vi "sv_Compute Time to Next Optimum for Sine Wave.vi"(7 "optimum":T1, 10 "phase (0 °)":dbl, 11 "frequency (997 Hz)":dbl) -> (3 "time to optimum [s]":dbl)   [LabVIEW 2017, in "SoundVib_Generation.lvlib"]
uses:
  <vilib>/addons/_NISVFA/_Generation/SoundVib_Generation.lvlib
  <vilib>/addons/_NISVFA/_Generation/subVIs/sv_Optimum Location.ctl
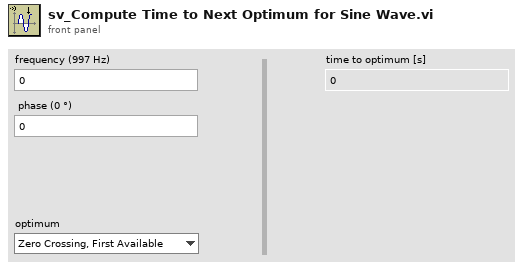
[diagram p1: front panel]
types:
  T1 = typedef "SoundVib_Generation.lvlib/sv_Optimum Location.ctl" = enum16{"Zero Crossing, First Available", "Zero Crossing, Positive Slope", "Zero Crossing, Negative Slope", "Peak or Valley", "Peak", "Valley"}
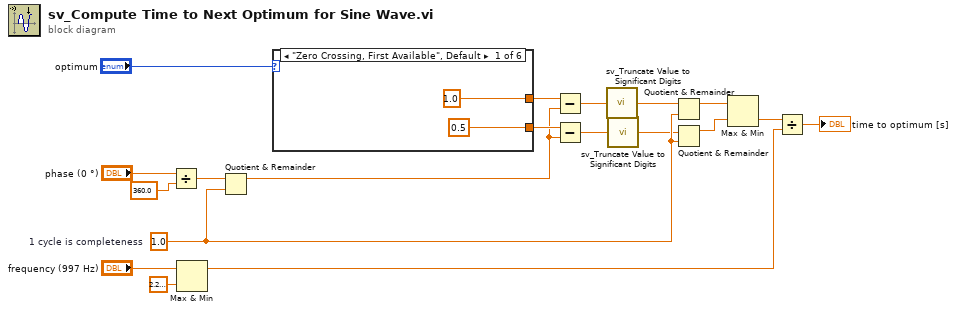
[diagram p0: block diagram]
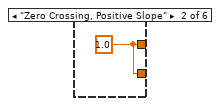
[diagram p2: hidden frame]
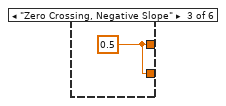
[diagram p3: hidden frame]
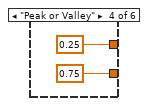
[diagram p4: hidden frame]
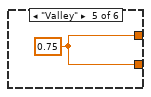
[diagram p5: hidden frame]
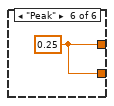
[diagram p6: hidden frame]
diagram:
  w8 = 1.0  # 1 cycle is completeness
  n1 = Divide(x="phase (0 °)", y=360.0 ("time to optimum [s]")) -> (x/y=w16:dbl)
  n2 = Max & Min(x="frequency (997 Hz)", y=2.220446049250313e-16) -> (max(x,y)=w11:dbl)  [unwired: 1 out]
  n3 = Quotient & Remainder(x=w16, y=w8) -> (x-y*floor(x/y)=w6:dbl)  [unwired: 1 out]
  n4 = case shown="\"Zero Crossing, First Available\", Default" "optimum" {
    tunnel: [1.0 ("time to optimum [s]") w22 w23 0.25 ("x") w26 w27] -> w10
    tunnel: [0.5 ("time to optimum [s]") w22 w23 0.75 ("x") w26 w27] -> w9
    frame "Zero Crossing, First Available", Default {
    }
    frame "Zero Crossing, Positive Slope" {
      w22 = 1.0 ("time to optimum [s]")
    }
    frame "Zero Crossing, Negative Slope" {
      w23 = 0.5 ("1 cycle is completeness")
    }
    frame "Peak or Valley" {
    }
    frame "Valley" {
      w26 = 0.75 ("x")
    }
    frame "Peak" {
      w27 = 0.25 ("x")
    }
  }
  n5 = Subtract(x=w10, y=w6) -> (x-y=w4:dbl)
  n6 = Subtract(x=w9, y=w6) -> (x-y=w2:dbl)
  n7 = call <vilib>:"sv_Truncate Value to Significant Digits.vi"("value"=w4) -> ("truncated value"=w3:dbl)  [unwired: 14 in]
  n8 = call <vilib>:"sv_Truncate Value to Significant Digits.vi"("value"=w2) -> ("truncated value"=w1:dbl)  [unwired: 14 in]
  n9 = Quotient & Remainder(x=w3, y=w8) -> (x-y*floor(x/y)=w15:dbl)  [unwired: 1 out]
  n10 = Quotient & Remainder(x=w1, y=w8) -> (x-y*floor(x/y)=w14:dbl)  [unwired: 1 out]
  n11 = Max & Min(x=w15, y=w14) -> (min(x,y)=w7:dbl)  [unwired: 1 out]
  n12 = Divide(x=w7, y=w11) -> (x/y=→"time to optimum [s]":dbl)
